vi "Example.vi"() -> ()   [LabVIEW 2012]
panel:
  out "Image 2":T1(plugin-control)
  out "Oil Value":sgl
  out "Water Value":sgl
  in  "Speed":u32=1000
  in  "stop":bool
  in  "Process Folder":path
  in  "TempFile":path
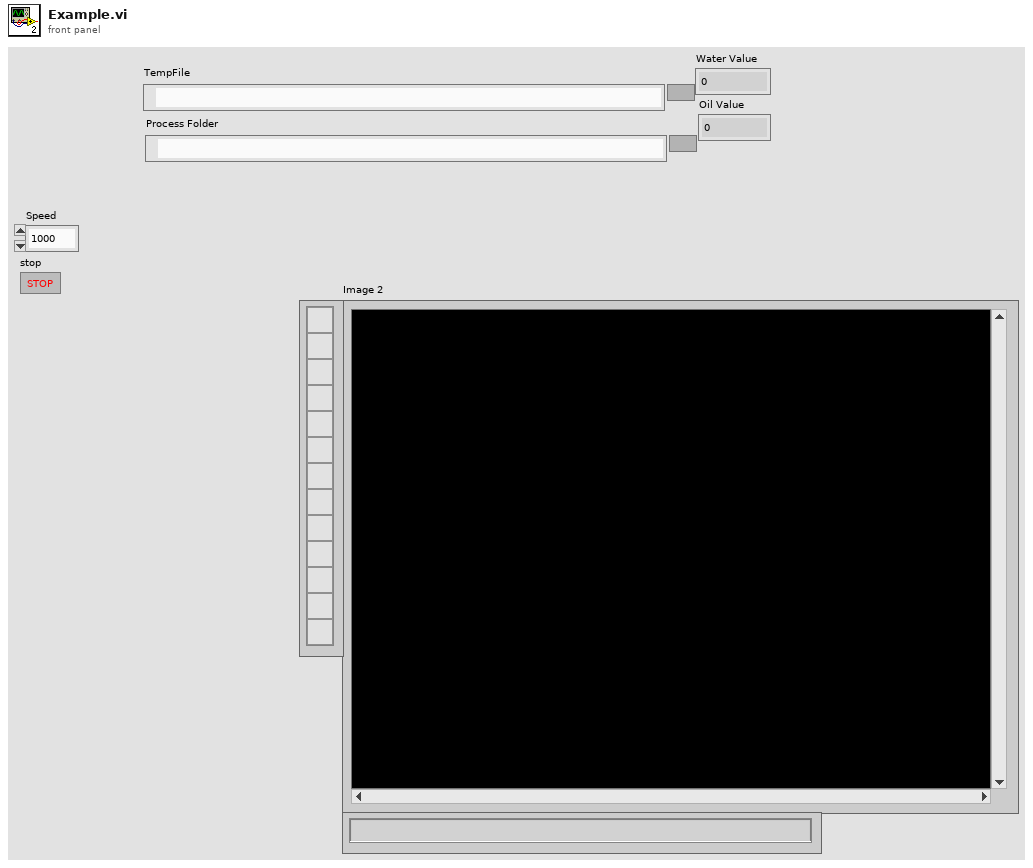
[diagram p1: front panel]
types:
  T1 = typedef "IMAQ Image.ctl" = refnum<image>
  T2 = typedef "imagedata.ctl" = cluster{"image type":i32, "image depth":i32, "image":u8[], "mask":u8[], "colors":u32[], "Rectangle":cluster{"left":i16, "top":i16, "right":i16, "bottom":i16}}
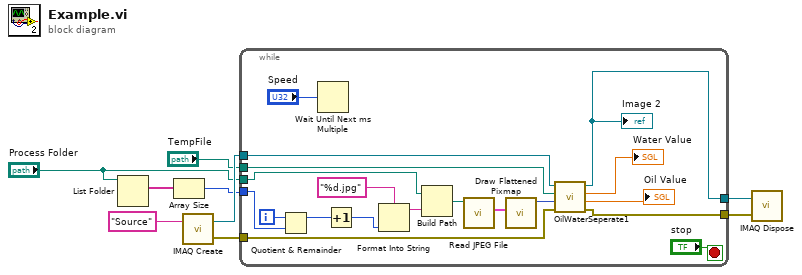
[diagram p0: block diagram]
diagram:
  n1 = List Folder(path="Process Folder") -> (filenames=w2:string[])  [unwired: 3 in, 3 out]
  n2 = Array Size(array=w2) -> (size(s)=w1:i32)
  n3 = call "IMAQ Create"("Image Name"="Source") -> ("New Image"=w9:T1, "error out"=w8:errorcluster)  [unwired: 4 in]
  n4 = while {
    tunnel: w9 -> [w28]
    tunnel: w8 -> [w27]
    tunnel: [w26] -> w6
    tunnel: [w10] -> w5
    tunnel: "TempFile" -> [w25]
    tunnel: "Process Folder" -> [w18]
    tunnel: w1 -> [w20]
    i -> [w14]
    stop <- "stop" stop-if-true
    n5 = Quotient & Remainder(x=w14, y=w20) -> (x-y*floor(x/y)=w15:i32)  [unwired: 1 out]
    n6 = Wait Until Next ms Multiple(millisecond multiple="Speed") -> ()  [unwired: 1 out]
    n7 = Increment(x=w15) -> (x+1=w13:i32)
    n8 = Format Into String(format string="%d.jpg", w13) -> (resulting string=w16:string)  [unwired: 2 in, 1 out]
    n9 = Build Path(base path=w18, name or relative path=w16) -> (appended path=w19:path)
    n10 = call <vilib>:"Read JPEG File.vi"("path to JPEG file"=w19) -> ("image data"=w24:T2)  [unwired: 8 in, 2 out]
    n11 = call <vilib>:"Draw Flattened Pixmap.vi"("image data"=w24) -> ("new picture"=w23:picture)  [unwired: 8 in]
    n12 = call "OilWaterSeperate1.vi"("error in (no error)"=w27, "2D Picture"=w23, "Temp path"=w25, "Image in"=w28) -> ("error out"=w26:errorcluster, "Oil Value"=→"Oil Value":sgl, "Water Value"=→"Water Value":sgl, "Image Out"=w10:T1)  [unwired: 4 in]
    "Image 2" <- w10
  }
  n13 = call "IMAQ Dispose"("Image"=w5, "error in (no error)"=w6) -> ()  [unwired: 4 in, 1 out]
